vi "UserInterfaceEventPattern 1.vi"() -> ()   [LabVIEW 2018]
doc: "Use this template to build a user interface event handler design pattern. Use this pattern for dialog boxes and other user interfaces. You also can create and execute user-defined events that the VI can handle the same way as user interface events."
panel:
  out "x+1":i32
  out "data out":string
  in  "Button 1":bool
  in  "stop":bool
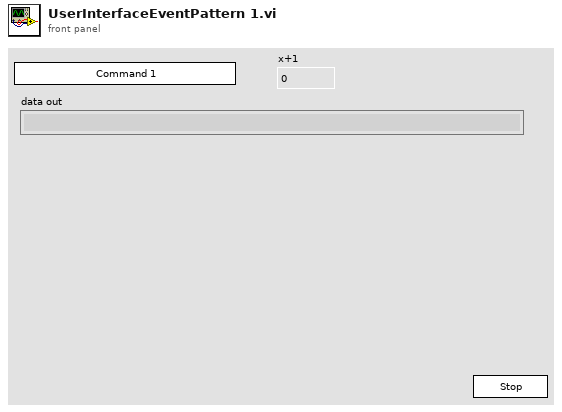
[diagram p1: front panel]
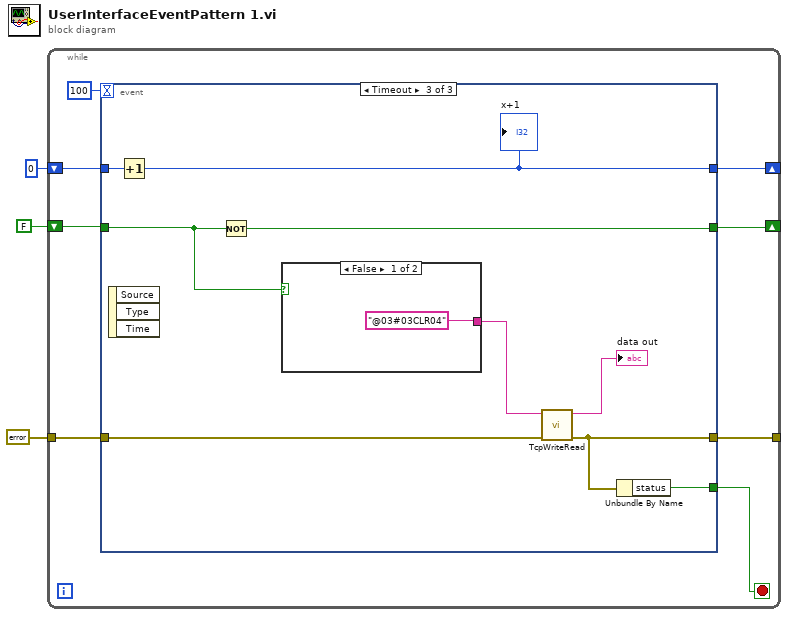
[diagram p0: block diagram]
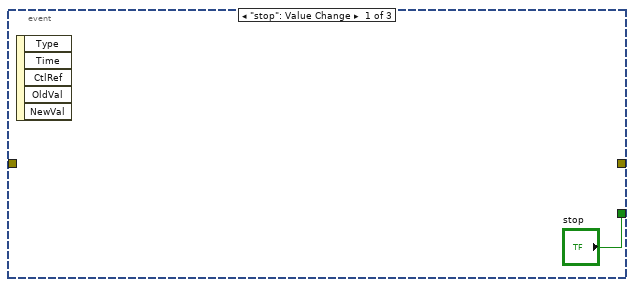
[diagram p2: hidden frame]
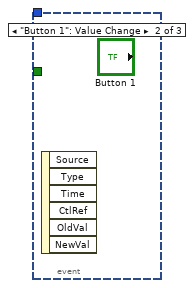
[diagram p3: hidden frame]
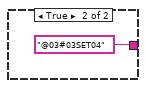
[diagram p4: hidden frame]
diagram:
  n1 = while {
    shift-right: [w9] -> _
    shift-left: FALSE -> [w8]
    tunnel: errorcluster {"status"=FALSE, "code"=0, "source"=""} ("error in") -> [w7]
    tunnel: [w6] -> _
    shift-right: [w4] -> _
    shift-left: 0 -> [w5]
    stop <- w11 stop-if-true
    n2 = event shown="[2] Timeout" {
      selector: _ -> [_ _ _]
      dyn-events: _ -> [_ _ _]
      timeout: 100 -> [_ _ _]
      tunnel: ["stop" _ w18] -> w11
      tunnel: w8 -> [_ _ w14]
      tunnel: [_ _ w13] -> w9
      tunnel: w7 -> [_ _ w20]
      tunnel: [_ _ w19] -> w6
      tunnel: w5 -> [_ _ w16]
      tunnel: [_ _ w15] -> w4
      event "stop": Value Change {
        n3 = event-data() -> ()  [unwired: 1 in, 5 out]
      }
      event "Button 1": Value Change {
        n4 = event-data() -> ()  [unwired: 1 in, 6 out]
      }
      event Timeout {
        n5 = event-data() -> ()  [unwired: 1 in, 3 out]
        n6 = Increment(x=w16) -> (x+1=w15:i32)
        "x+1" <- w15
        n7 = Not(x=w14) -> (.not. x?=w13:bool)
        n8 = case shown="False" w14 {
          tunnel: ["@03#03CLR04" ("data in") "@03#03SET04" ("data in")] -> w21
          frame False {
          }
          frame True {
          }
        }
        n9 = call "TcpWriteRead.vi"("error in"=w20, "data in"=w21) -> ("error out"=w19:errorcluster, "data out"=→"data out":string)  [unwired: 8 in]
        n10 = Unbundle By Name(w19) -> ("status"=w18:bool)
      }
    }
  }
